vi "Reciev_CANATII - Mod.vi"(0 "Config":refnum<vi>, 2 "queue out":refnum<queue>, 5 "cnd_in":u32) -> (4 "str out":string, 6 "cnt_out":u32, 7 "queue out 2":refnum<queue>, 8 "Data":u8[](array[numeric]))   [LabVIEW 2017]
uses:
  PCAN_Driver/ControlCAN.lvlib
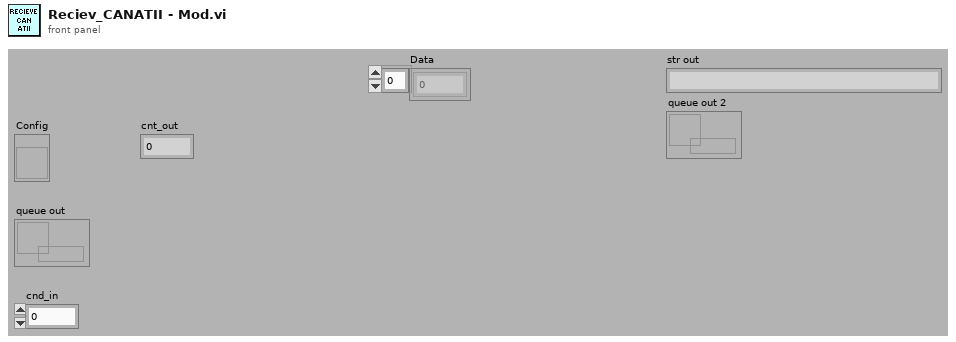
[diagram p1: front panel]
types:
  T1 = typedef "ControlCAN.lvlib/DevType.ctl" = u32
  T2 = typedef "ControlCAN.lvlib/CAN Channel.ctl" = u32
  T3 = typedef "ControlCAN.lvlib/VCI_INIT_CONFIG.ctl" = cluster{"AccCode":u32, "AccMask":u32, "InitFlag":T4, "Fliter":T5, "Timing0":u8, "Timing1":u8, "Mode":T6}
  T4 = typedef "ControlCAN.lvlib/InitFlag.ctl" = u32
  T5 = typedef "ControlCAN.lvlib/Fliter.ctl" = u8
  T6 = typedef "ControlCAN.lvlib/Mode.ctl" = u8
  T7 = cluster{"DevType":T1, "DevIndex":u32, "CanIndex":T2, "VCI_INIT_CONFIG":T3}
  T8 = typedef "ControlCAN.lvlib/VCI_CAN_OBJ.ctl" = cluster{"ID":u32, "TimeStamp":u32, "TimeFlag":u8, "SendType":u8, "RemoteFlag":u8, "ExternFlag":u8, "DataLen":u8, "Data":u8[], "Reserved":u8[]}
  T9 = cluster{"ID":u32, "MSGTYPE":u8, "LEN":u8, "aDATA":u8[]}
  T10 = cluster{"Type":enum16{"接收", "发送"}, "Channel":T2, "Time":timestamp, "VCI_CAN_OBJ":T8}[]
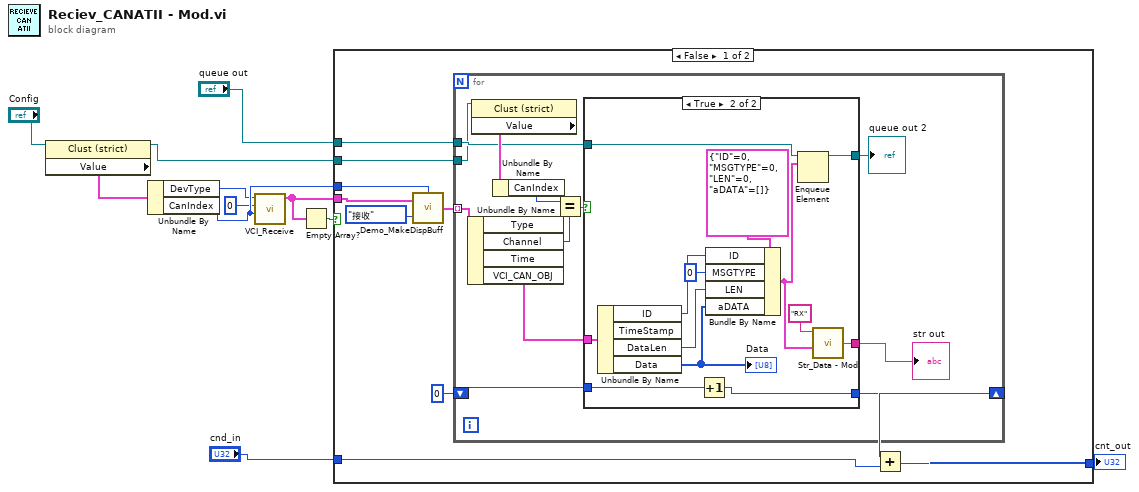
[diagram p0: block diagram]
diagram:
  n1 = property class="Clust (strict)"(reference="Config") -> (reference out=w1:refnum<vi>, "Value"=w8:T7)  [unwired: 1 in, 1 out]
  n2 = Unbundle By Name(w8) -> ("DevType"=w6:T1, "CanIndex"=w7:T2)
  n3 = call "VCI_Receive.vi"("CANIndex"=w7, "DevIndex"=u32 0, "DevType"=w6) -> ("Recieve"=w5:T8[])  [unwired: 3 in, 5 out]
  n4 = Empty Array?(array=w5) -> (empty?=w4:bool)
  n5 = case shown="False" w4 {
    tunnel: w5 -> [w19 _]
    tunnel: w7 -> [w20 _]
    tunnel: "cnd_in" -> [w15 w49]
    tunnel: [w14 w49] -> w9
    tunnel: "queue out" -> [w13 _]
    tunnel: w1 -> [w12 _]
    frame False {
      n6 = call "Demo_MakeDispBuff.vi"("Channel"=w20, "Type"=enum16{"接收", "发送"}."接收", "OBJs"=w19) -> ("Buffer"=w18:T10)
      n7 = for {
        tunnel: w18 -> [w33] mode=indexing
        tunnel: w13 -> [w25]
        shift-right: [w26] -> w16
        shift-left: u32 0 -> [w27]
        tunnel: w12 -> [w24]
        n8 = Unbundle By Name(w33) -> ("Channel"=w29:T2, "VCI_CAN_OBJ"=w32:T8)  [unwired: 2 out]
        n9 = property class="Clust (strict)"(reference=w24) -> ("Value"=w31:T7)  [unwired: 1 in, 2 out]
        n10 = Unbundle By Name(w31) -> ("CanIndex"=w30:T2)
        n11 = Equal?(x=w30, y=w29) -> (x = y?=w28:bool)
        n12 = case shown="True" w28 {
          tunnel: w25 -> [w34 w41]
          tunnel: w32 -> [_ w47]
          tunnel: w27 -> [w35 w43]
          tunnel: [w35 w42] -> w26
          tunnel: [w34 w37] -> w23
          tunnel: [_ w36] -> w22
          frame False {
          }
          frame True {
            n13 = Unbundle By Name(w47) -> ("ID"=w46:u32, "DataLen"=w45:u8, "Data"=w44:u8[])  [unwired: 1 out]
            "Data" <- w44
            n14 = Increment(x=w43) -> (x+1=w42:u32)
            n15 = Bundle By Name(cluster=T9 {"ID"=0, "MSGTYPE"=0, "LEN"=0, "aDATA"=[]} ("Msg"), "ID"=w46, "MSGTYPE"=u8 0, "LEN"=w45, "aDATA"=w44) -> (w39:T9)
            n16 = Enqueue Element(queue=w41, element=w39) -> (queue out=w37:refnum<queue>)  [unwired: 1 in, 3 out]
            n17 = call "Str_Data - Mod.vi"("Msg"=w39, "string"="RX") -> ("str out"=w36:string)  [unwired: 4 in]
          }
        }
        "str out" <- w22
        "queue out 2" <- w23
      }
      n18 = Add(x=w16, y=w15) -> (x+y=w14:u32)
    }
    frame True {
    }
  }
  "cnt_out" <- w9
